vi "AlliGator Python Plugin Get Function Name.vi"(8 "Error In":errorcluster, 9 "Source":string, 11 "String in":string) -> (0 "Error Out":errorcluster, 1 "function_name":string, 2 "Is preceded by Separator":bool, 3 "String out":string)   [LabVIEW 2021, in "AlliGator Python Plugins.lvlib"]
doc: "Returns function name and whether the function should be preceded by a separator in the menu."
uses:
  AlliGator Python Plugins.lvlib
  <userlib>/_OpenG.lib/string/string.llb/openg_string.lvlib
panel:
  # "see the AlliGator License on the block diagram (Ctrl+E or Window:Show Block Diagram)"
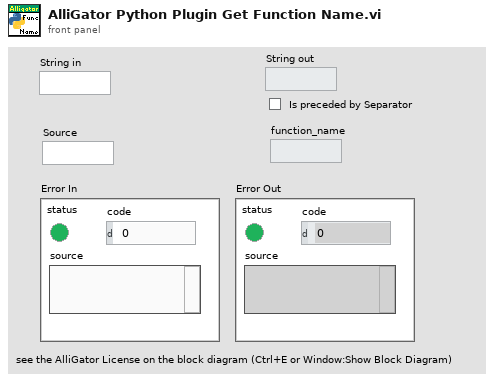
[diagram p1: front panel]
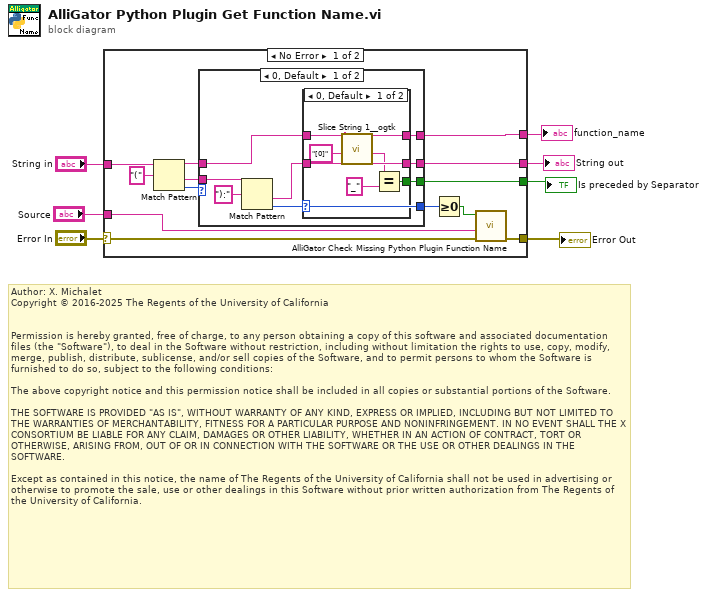
[diagram p0: block diagram]
diagram:
  # "Author: X. Michalet\nCopyright © 2016-2025 The Regents of the University of California\n \n\nPermission is hereby granted, free of charge, to any person obtaining a copy of this software and associated documentation files (the \"Software\"), to deal in the Software without restriction, including without limitation the rights to use, copy, modify, merge, publish, distribute, sublicense, and/or sell copies of the Software, and to permit persons to whom the Software is furnished to do so, subject to the following conditions:\n\nThe above copyright notice and this permission notice shall be included in all copies or substantial portions of the Software.\n\nTHE SOFTWARE IS PROVIDED \"AS IS\", WITHOUT WARRANTY OF ANY KIND, EXPRESS OR IMPLIED, INCLUDING BUT NOT LIMITED TO THE WARRANTIES OF MERCHANTABILITY, FITNESS FOR A PARTICULAR PURPOSE AND NONINFRINGEMENT. IN NO EVENT SHALL THE X CONSORTIUM BE LIABLE FOR ANY CLAIM, DAMAGES OR OTHER LIABILITY, WHETHER IN AN ACTION OF CONTRACT, TORT OR OTHERWISE, ARISING FROM, OUT OF OR IN CONNECTION WITH THE SOFTWARE OR THE USE OR OTHER DEALINGS IN THE SOFTWARE.\n\nExcept as contained in this notice, the name of The Regents of the University of California shall not be used in advertising or otherwise to promote the sale, use or other dealings in this Software without prior written authorization from The Regents of the University of California."
  n1 = case shown="No Error" "Error In" {
    selector: "Error In" -> [w13 w38]
    tunnel: [w20 w39] -> w7
    tunnel: "String in" -> [w18 w39]
    tunnel: [w14 _] -> w5
    tunnel: [w11 w38] -> w3
    tunnel: "Source" -> [w12 _]
    tunnel: [w8 _] -> w1
    frame No Error {
      n2 = Match Pattern(string=w18, regular expression="(") -> (before substring=w15:string, after substring=w19:string, offset past match=w16:i32)  [unwired: 1 in, 1 out]
      n3 = case shown="0, Default" w16 {
        selector: w16 -> [_ w36]
        tunnel: [w24 w37] -> w20
        tunnel: w19 -> [w27 _]
        tunnel: w15 -> [w25 w37]
        tunnel: [w23 _] -> w14
        tunnel: [w22 w36] -> w10
        tunnel: [w21 _] -> w8
        frame 0, Default {
          n4 = Match Pattern(string=w27, regular expression="):") -> (after substring=w26:string, offset past match=w22:i32)  [unwired: 1 in, 2 out]
          n5 = case shown="0, Default" w22 {
            tunnel: w26 -> [w34 _]
            tunnel: w25 -> [w33 w35]
            tunnel: [w34 w35] -> w24
            tunnel: [w33 _] -> w23
            tunnel: [w29 _] -> w21
            frame 0, Default {
              n6 = call <userlib>:"Slice String 1__ogtk.vi"("Subset (i:j)"="[0]", "String"=w33) -> ("Substring (String[i:j])"=w31:string)  [unwired: 7 in]
              n7 = Equal?(x=w31, y="_") -> (x = y?=w29:bool)
            }
            frame -1 {
            }
          }
        }
        frame -1 {
        }
      }
      n8 = Greater Or Equal To 0?(x=w10) -> (x >= 0?=w9:bool)
      n9 = call "AlliGator Check Missing Python Plugin Function Name.vi"("error in (no error)"=w13, "Source"=w12, "Function Name Found"=w9) -> ("error out"=w11:errorcluster)  [unwired: 8 in]
    }
    frame Error {
    }
  }
  "String out" <- w7
  "function_name" <- w5
  "Error Out" <- w3
  "Is preceded by Separator" <- w1
